vi "Aq Read.vi"(8 "error in (no error)":errorcluster, 11 "VISA resource name":refnum<visa-resource-name>) -> (0 "error out":errorcluster, 2 "Imag Data":i32[](array[numeric]), 3 "Real Data":i32[](array[numeric]))   [LabVIEW 2011]
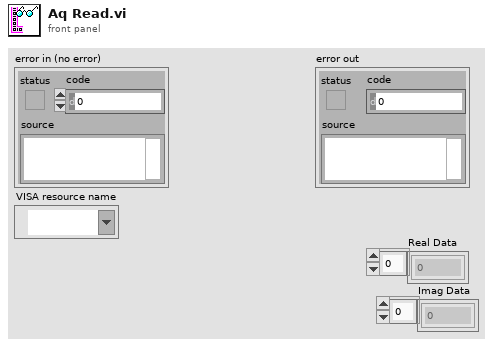
[diagram p1: front panel]
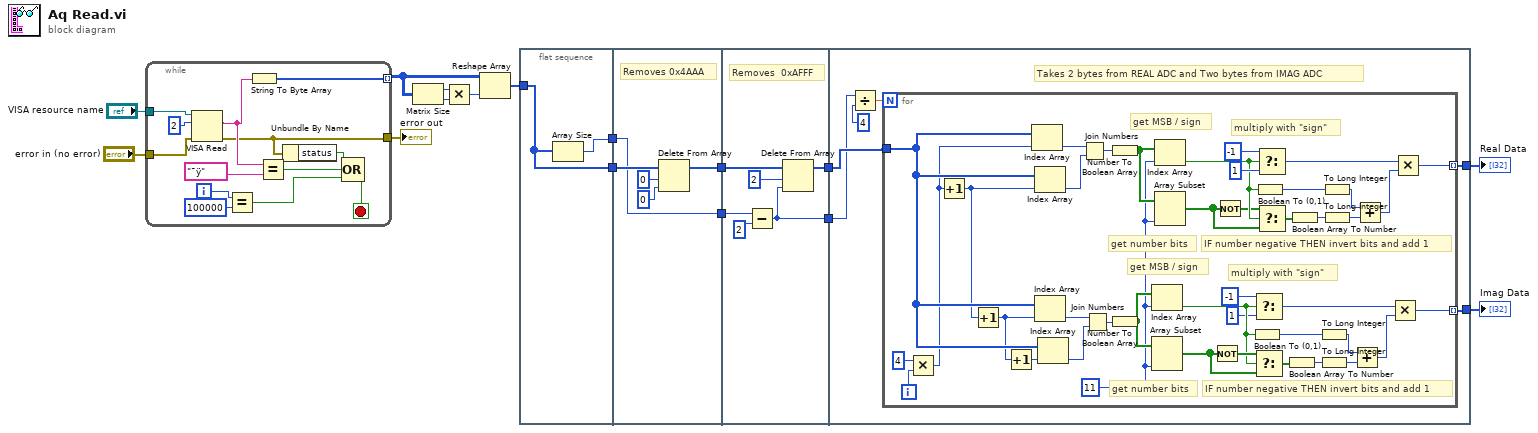
[diagram p0: block diagram]
diagram:
  n1 = while {
    tunnel: [w29] -> w16 mode=indexing
    tunnel: "error in (no error)" -> [w19]
    tunnel: [w18] -> w2
    tunnel: "VISA resource name" -> [w17]
    i -> [w26]
    stop <- w22 stop-if-true
    n2 = VISA Read(VISA resource name=w17, byte count=u32 2, error in (no error)=w19) -> (read buffer=w20:string, error out=w18:errorcluster)  [unwired: 2 out]
    n3 = Equal?(x=w26, y=100000) -> (x = y?=w23:bool)
    n4 = String To Byte Array(string=w20) -> (unsigned byte array=w29:u8[])
    n5 = Equal?(x=w20, y="¯ÿ" ("search string/char (-)")) -> (x = y?=w24:bool)
    n6 = Unbundle By Name(w18) -> ("status"=w21:bool)
    n7 = Compound Arithmetic op=OR(w21, w24, w23) -> (w22:bool)
  }
  "error out" <- w2
  n8 = Matrix Size(0:w16) -> (1:w14:i32, 2:w15:i32)
  n9 = Multiply(x=w14, y=w15) -> (x*y=w13:i32)
  n10 = Reshape Array(w16, w13) -> (w6:u8[])
  n11 = flat-sequence {
    tunnel: [w31] -> w12
    tunnel: [w30] -> w11
    tunnel: w6 -> [w31]
    tunnel: w12 -> [w36]
    tunnel: w11 -> [w32]
    tunnel: [w34] -> w10
    tunnel: [w32] -> w9
    tunnel: w10 -> [w42]
    tunnel: w9 -> [w38]
    tunnel: [w40] -> w8
    tunnel: [w37] -> w7
    tunnel: w8 -> [w48]
    tunnel: [w47] -> w5
    tunnel: [w46] -> w4
    tunnel: w7 -> [w44]
    frame #0 {
      n12 = Array Size(array=w31) -> (size(s)=w30:i32)
    }
    frame #1 {
      # "Removes 0x4AAA"
      n13 = Delete From Array(array=w36, length=0, index=0) -> (array with subset deleted=w34:u8[])  [unwired: 1 out]
    }
    frame #2 {
      # "Removes  0xAFFF"
      n14 = Subtract(x=w38, y=2 ("length")) -> (x-y=w37:i32)
      n15 = Delete From Array(array=w42, length=2, index=w37) -> (array with subset deleted=w40:u8[])  [unwired: 1 out]
    }
    frame #3 {
      # "Takes 2 bytes from REAL ADC and Two bytes from IMAG ADC"
      n16 = Divide(x=w44, y=4) -> (x/y=w43:dbl)
      n17 = for {
        N: w43 -> [_]
        tunnel: w48 -> [w85]
        tunnel: [w64] -> w47 mode=indexing
        tunnel: [w50] -> w46 mode=indexing
        i -> [w82]
        w49 = 11 ("length")
        # "multiply with \"sign\""
        # "IF number negative THEN invert bits and add 1"
        # "get number bits"
        # "get MSB / sign"
        # "multiply with \"sign\""
        # "IF number negative THEN invert bits and add 1"
        # "get number bits"
        # "get MSB / sign"
        n18 = Multiply(x=4, y=w82) -> (x*y=w80:i32)
        n19 = Increment(x=w80) -> (x+1=w83:i32)
        n20 = Increment(x=w83) -> (x+1=w84:i32)
        n21 = Increment(x=w84) -> (x+1=w86:i32)
        n22 = Index Array(array=w85, index=w80) -> (element=w90:u8)
        n23 = Index Array(array=w85, index=w83) -> (element=w89:u8)
        n24 = Index Array(array=w85, index=w84) -> (element=w87:u8)
        n25 = Index Array(array=w85, index=w86) -> (element=w88:u8)
        n26 = Join Numbers(hi=w90, lo=w89) -> ((hi.lo)=w78:u16)
        n27 = Join Numbers(hi=w87, lo=w88) -> ((hi.lo)=w79:u16)
        n28 = Number To Boolean Array(number=w78) -> (Boolean array=w65:bool[])
        n29 = Number To Boolean Array(number=w79) -> (Boolean array=w51:bool[])
        n30 = Index Array(array=w51, index=w49) -> (element=w57:bool)
        n31 = Array Subset(array=w51, length=w49) -> (w61:bool[])  [unwired: 1 in]
        n32 = Index Array(array=w65, index=w49) -> (element=w72:bool)
        n33 = Array Subset(array=w65, length=w49) -> (w68:bool[])  [unwired: 1 in]
        n34 = Not(x=w61) -> (.not. x?=w62:bool[])
        n35 = Not(x=w68) -> (.not. x?=w67:bool[])
        n36 = Boolean To (0,1)(Boolean=w57) -> (0, 1=w58:i16)
        n37 = Select(t=-1, s=w57, f=1) -> (s? t:f=w54:i32)
        n38 = Select(t=w62, s=w57, f=w61) -> (s? t:f=w60:bool[])
        n39 = Boolean To (0,1)(Boolean=w72) -> (0, 1=w71:i16)
        n40 = Select(t=-1, s=w72, f=1) -> (s? t:f=w75:i32)
        n41 = Select(t=w67, s=w72, f=w68) -> (s? t:f=w69:bool[])
        n42 = Boolean Array To Number(Boolean array=w60) -> (number=w63:u32)
        n43 = Boolean Array To Number(Boolean array=w69) -> (number=w66:u32)
        n44 = To Long Integer(number=w58) -> (32bit integer=w52:i32)
        n45 = To Long Integer(number=w63) -> (32bit integer=w59:i32)
        n46 = To Long Integer(number=w71) -> (32bit integer=w77:i32)
        n47 = To Long Integer(number=w66) -> (32bit integer=w70:i32)
        n48 = Add(x=w52, y=w59) -> (x+y=w53:i32)
        n49 = Add(x=w77, y=w70) -> (x+y=w76:i32)
        n50 = Multiply(x=w54, y=w53) -> (x*y=w50:i32)
        n51 = Multiply(x=w75, y=w76) -> (x*y=w64:i32)
      }
    }
  }
  "Real Data" <- w5
  "Imag Data" <- w4
